vi "Select_List.vi"(7 "Load ERD List":T2) -> (8 "ERD Read List":T1(array[cluster])=[{"Boolean"=TRUE, "ERD Number"=49, "ERD Name"="Build Number", "Data Type"=enum."uint32_t"}, {"Boolean"=TRUE, "ERD Number"=127, "ERD Name"="Build Hash", "Data Type"=enum."string"}, {"Boolean"=TRUE, "ERD Number"=61467, "ERD Name"="Machine State", "Data Type"=enum."uint8_t"}, {"Boolean"=TRUE, "ERD Number"=61457, "ERD Name"="Relay Status", "Data Type"=enum."string"}, {"Boolean"=TRUE, "ERD Number"=61459, "ERD Name"="Door Switch State", "Data Type"=enum."string"}, {"Boolean"=TRUE, "ERD Number"=61460, "ERD Name"="Door Latch State", "Data Type"=enum."string"}, {"Boolean"=TRUE, "ERD Number"=61461, "ERD Name"="Inlet Thermistor", "Data Type"=enum."uint16_t"}, {"Boolean"=TRUE, "ERD Number"=61462, "ERD Name"="Outlet Thermistor", "Data Type"=enum."uint16_t"}, {"Boolean"=TRUE, "ERD Number"=61468, "ERD Name"="Control Lock State", "Data Type"=enum."string"}, {"Boolean"=TRUE, "ERD Number"=61483, "ERD Name"="Signal Volume", "Data Type"=enum."string"}, {"Boolean"=TRUE, "ERD Number"=61582, "ERD Name"="Drum Light", "Data Type"=enum."string"}, {"Boolean"=TRUE, "ERD Number"=61478, "ERD Name"="Delay Time", "Data Type"=enum."string"}, {"Boolean"=TRUE, "ERD Number"=8275, "ERD Name"="Ext. Tumble", "Data Type"=enum."string"}, {"Boolean"=TRUE, "ERD Number"=61480, "ERD Name"="Sub Cycle", "Data Type"=enum."uint8_t"}, {"Boolean"=TRUE, "ERD Number"=8272, "ERD Name"="Temp Level", "Data Type"=enum."string"}, {"Boolean"=TRUE, "ERD Number"=8269, "ERD Name"="Dryness Level", "Data Type"=enum."string"}, {"Boolean"=TRUE, "ERD Number"=8262, "ERD Name"="eDry", "Data Type"=enum."string"}, {"Boolean"=TRUE, "ERD Number"=61495, "ERD Name"="Time Level", "Data Type"=enum."string"}, {"Boolean"=TRUE, "ERD Number"=8266, "ERD Name"="Damp Alert", "Data Type"=enum."string"}, {"Boolean"=TRUE, "ERD Number"=61501, "ERD Name"="Detangle", "Data Type"=enum."string"}, {"Boolean"=TRUE, "ERD Number"=61510, "ERD Name"="MyCycle", "Data Type"=enum."string"}, {"Boolean"=TRUE, "ERD Number"=61594, "ERD Name"="Cycle Engine State", "Data Type"=enum."string"}, {"Boolean"=TRUE, "ERD Number"=61597, "ERD Name"="Cycle Selected", "Data Type"=enum."string"}, {"Boolean"=TRUE, "ERD Number"=61443, "ERD Name"="Tune ID", "Data Type"=enum."string"}, {"Boolean"=TRUE, "ERD Number"=61503, "ERD Name"="Delay Option", "Data Type"=enum."string"}, {"Boolean"=TRUE, "ERD Number"=61619, "ERD Name"="Restriction Detection Status", "Data Type"=enum."string"}, {"Boolean"=TRUE, "ERD Number"=61618, "ERD Name"="Vent Restriction", "Data Type"=enum."string"}, {"Boolean"=TRUE, "ERD Number"=61611, "ERD Name"="Load Size By Contact", "Data Type"=enum."string"}, {"Boolean"=TRUE, "ERD Number"=61613, "ERD Name"="Load Size by Temp", "Data Type"=enum."string"}, {"Boolean"=TRUE, "ERD Number"=61615, "ERD Name"="LoadSizeByAggregation", "Data Type"=enum."string"}, {"Boolean"=TRUE, "ERD Number"=61605, "ERD Name"="Sensor Dry Status", "Data Type"=enum."string"}, {"Boolean"=TRUE, "ERD Number"=61626, "ERD Name"="Check Dampness State", "Data Type"=enum."string"}, {"Boolean"=TRUE, "ERD Number"=61624, "ERD Name"="MoistureSensorRawAdcFromMc", "Data Type"=enum."string"}, {"Boolean"=TRUE, "ERD Number"=62242, "ERD Name"="SmoothMoistureReading", "Data Type"=enum."string"}, {"Boolean"=TRUE, "ERD Number"=61463, "ERD Name"="Filtered Moisture", "Data Type"=enum."string"}, {"Boolean"=TRUE, "ERD Number"=61608, "ERD Name"="TargetMoistureVoltage", "Data Type"=enum."string"}, {"Boolean"=TRUE, "ERD Number"=61609, "ERD Name"="TargetMoistureVoltageReached", "Data Type"=enum."string"}, {"Boolean"=TRUE, "ERD Number"=61719, "ERD Name"="MaxFilteredMoistureVoltageDuringASensingCycle", "Data Type"=enum."string"}, {"Boolean"=TRUE, "ERD Number"=61555, "ERD Name"="TrimmerBothCoilInhibitRequest", "Data Type"=enum."string"}, {"Boolean"=TRUE, "ERD Number"=61567, "ERD Name"="TrimmerInhibitRelay1", "Data Type"=enum."string"}, {"Boolean"=TRUE, "ERD Number"=61568, "ERD Name"="TrimmerInhibitRelay2", "Data Type"=enum."string"}, {"Boolean"=TRUE, "ERD Number"=61549, "ERD Name"="HeatControlParametricData", "Data Type"=enum."string"}, {"Boolean"=TRUE, "ERD Number"=61610, "ERD Name"="EOC Reason", "Data Type"=enum."string"}, {"Boolean"=TRUE, "ERD Number"=61600, "ERD Name"="Heat Control Request", "Data Type"=enum."string"}, {"Boolean"=TRUE, "ERD Number"=61677, "ERD Name"="CoolDownStepStatus", "Data Type"=enum."string"}, {"Boolean"=TRUE, "ERD Number"=61554, "ERD Name"="OverTempHeaterInhibitRequest", "Data Type"=enum."string"}, {"Boolean"=TRUE, "ERD Number"=61565, "ERD Name"="EcoDryInhibitRelay1", "Data Type"=enum."string"}, {"Boolean"=TRUE, "ERD Number"=61566, "ERD Name"="EcoDryInhibitRelay2", "Data Type"=enum."string"}, {"Boolean"=TRUE, "ERD Number"=61743, "ERD Name"="ReverseDrumInhibitRelay1", "Data Type"=enum."string"}, {"Boolean"=TRUE, "ERD Number"=61744, "ERD Name"="ReverseDrumInhibitRelay2", "Data Type"=enum."string"}, {"Boolean"=TRUE, "ERD Number"=61556, "ERD Name"="NormalHeatControlMethodStatus", "Data Type"=enum."string"}, {"Boolean"=TRUE, "ERD Number"=61557, "ERD Name"="FallbackHeatControlMethodStatus", "Data Type"=enum."string"}, {"Boolean"=TRUE, "ERD Number"=61479, "ERD Name"="Remaining Cycle Time", "Data Type"=enum."string"}, {"Boolean"=TRUE, "ERD Number"=61698, "ERD Name"="InitialHeatingCycleTimeSeconds", "Data Type"=enum."string"}, {"Boolean"=TRUE, "ERD Number"=62214, "ERD Name"="InletTemperatureRawAdc\n", "Data Type"=enum."string"}, {"Boolean"=TRUE, "ERD Number"=62215, "ERD Name"="OutletTemperatureRawAdc", "Data Type"=enum."string"}, {"Boolean"=TRUE, "ERD Number"=61607, "ERD Name"="SensingCycleTotalDryingTimeSeconds", "Data Type"=enum."string"}, {"Boolean"=TRUE, "ERD Number"=61563, "ERD Name"="TimedCycleTotalDryingTimeSeconds", "Data Type"=enum."string"}, {"Boolean"=TRUE, "ERD Number"=61628, "ERD Name"="TimeToReachTargetVoltageSeconds", "Data Type"=enum."string"}, {"Boolean"=TRUE, "ERD Number"=61617, "ERD Name"="Dry Load Detection", "Data Type"=enum."string"}, {"Boolean"=TRUE, "ERD Number"=63510, "ERD Name"="Sensor DryTemp Multiplier 100", "Data Type"=enum."string"}, {"Boolean"=TRUE, "ERD Number"=61728, "ERD Name"="Erd_EcoDrySensorDryProfileSelectorStatus", "Data Type"=enum."string"}, {"Boolean"=TRUE, "ERD Number"=61729, "ERD Name"="Erd_EcoDrySensorDryProfileSelectorResultmeInSeconds", "Data Type"=enum."string"}, {"Boolean"=TRUE, "ERD Number"=61736, "ERD Name"="Erd_EcoDryControllerStatus", "Data Type"=enum."string"}, {"Boolean"=TRUE, "ERD Number"=61737, "ERD Name"="Erd_EcoDryRelay1TimerData", "Data Type"=enum."string"}, {"Boolean"=TRUE, "ERD Number"=61738, "ERD Name"="Erd_EcoDryRelay2TimerData", "Data Type"=enum."string"}, {"Boolean"=TRUE, "ERD Number"=61739, "ERD Name"="Erd_EcoDryStage2TransitionTimeInSeconds", "Data Type"=enum."string"}, {"Boolean"=TRUE, "ERD Number"=61606, "ERD Name"="Erd_ElapsedCycleTimeSeconds2TransitionTimeInSeconds", "Data Type"=enum."string"}, {"Boolean"=TRUE, "ERD Number"=63489, "ERD Name"="SensorDryDampSmallRestrictionSmallLoad\natus", "Data Type"=enum."string"}] {"ERD Number" format="%.0x"})   [LabVIEW 2023]
uses:
  Common/type defs/Choose_ERD_List.ctl
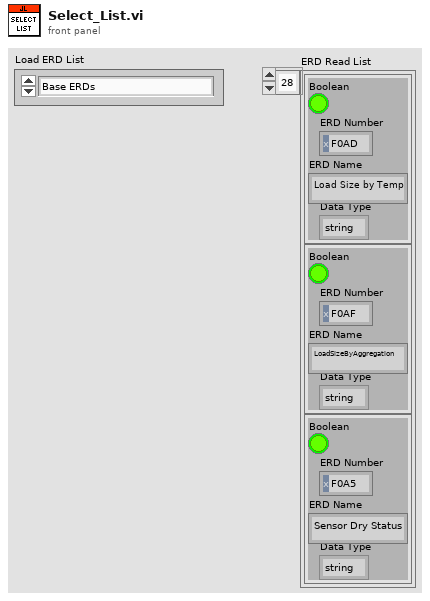
[diagram p1: front panel]
types:
  T1 = cluster{"Boolean":bool, "ERD Number":u16, "ERD Name":string, "Data Type":enum16{"string", "boolean", "uint8_t", "uint16_t", "uint32_t", "uint64_t", "int8_t", "int16_t", "int32_t", "int64_t"}}[]
  T2 = typedef "Choose_ERD_List.ctl" = enum16{"Base ERDs", "QA ERDs", "MABE ERD List", "EcoDry Evaluation ERD List", "ClothDampnessCheck ERD List"}
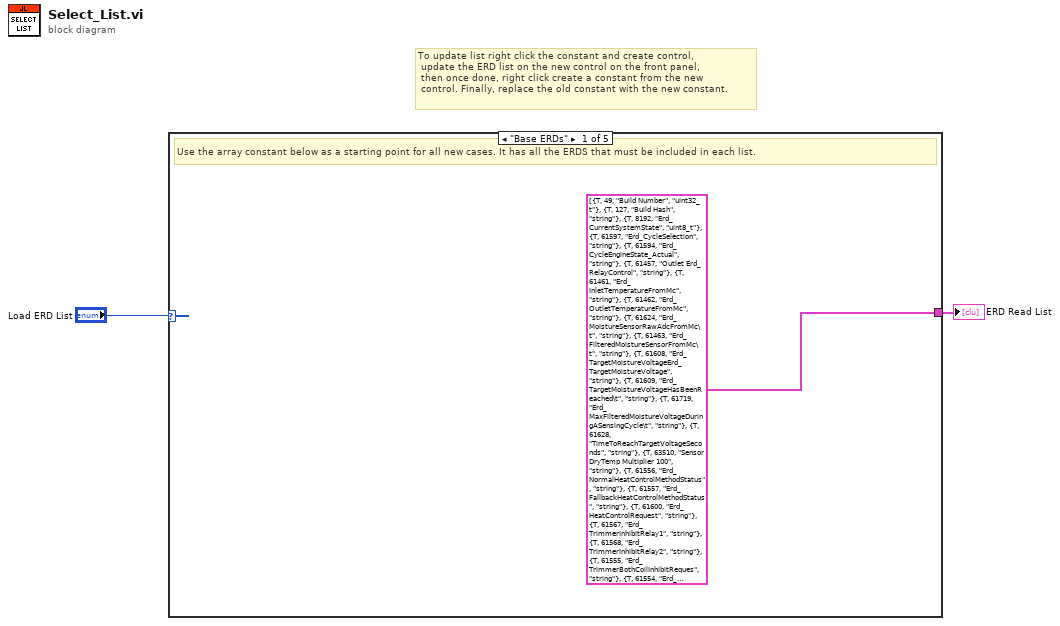
[diagram p0: block diagram]
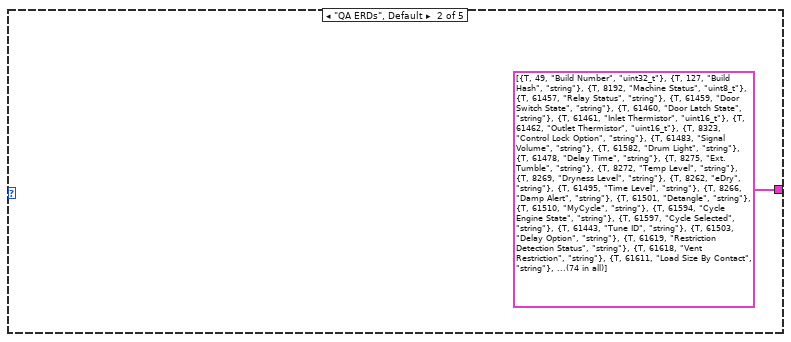
[diagram p2: hidden frame]
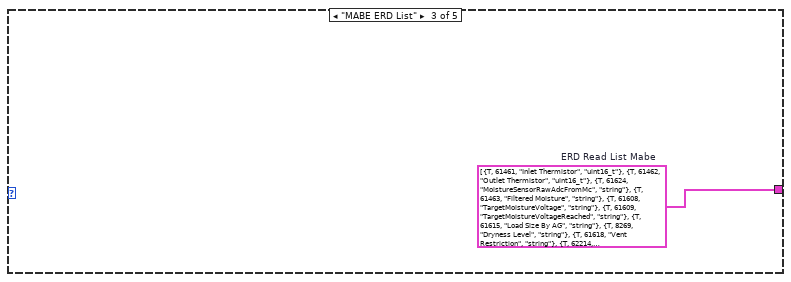
[diagram p3: hidden frame]
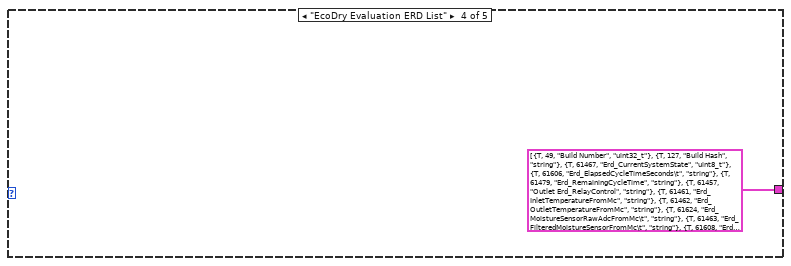
[diagram p4: hidden frame]
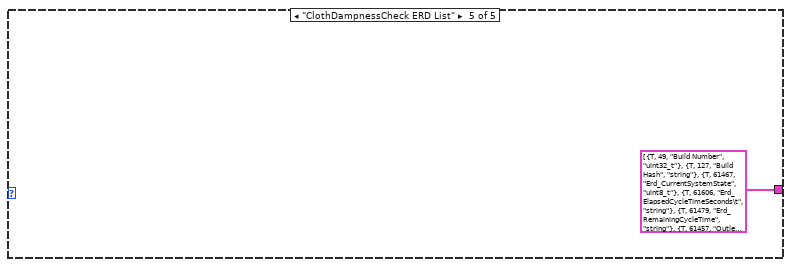
[diagram p5: hidden frame]
diagram:
  # "To update list right click the constant and create control,\n update the ERD list on the new control on the front panel,\n then once done, right click create a constant from the new\n control. Finally, replace the old constant with the new constant."
  n1 = case shown="\"Base ERDs\"" "Load ERD List" {
    tunnel: [T1 [{"Boolean"=TRUE, "ERD Number"=49, "ERD Name"="Build Number", "Data Type"=enum."uint32_t"}, {"Boolean"=TRUE, "ERD Number"=127, "ERD Name"="Build Hash", "Data Type"=enum."string"}, {"Boolean"=TRUE, "ERD Number"=8192, "ERD Name"="Erd_CurrentSystemState", "Data Type"=enum."uint8_t"}, {"Boolean"=TRUE, "ERD Number"=61597, "ERD Name"="Erd_CycleSelection", "Data Type"=enum."string"}, {"Boolean"=TRUE, "ERD Number"=61594, "ERD Name"="Erd_CycleEngineState_Actual", "Data Type"=enum."string"}, {"Boolean"=TRUE, "ERD Number"=61457, "ERD Name"="Outlet Erd_RelayControl", "Data Type"=enum."string"}, {"Boolean"=TRUE, "ERD Number"=61461, "ERD Name"="Erd_InletTemperatureFromMc", "Data Type"=enum."string"}, {"Boolean"=TRUE, "ERD Number"=61462, "ERD Name"="Erd_OutletTemperatureFromMc", "Data Type"=enum."string"}, {"Boolean"=TRUE, "ERD Number"=61624, "ERD Name"="Erd_MoistureSensorRawAdcFromMc\t", "Data Type"=enum."string"}, {"Boolean"=TRUE, "ERD Number"=61463, "ERD Name"="Erd_FilteredMoistureSensorFromMc\t", "Data Type"=enum."string"}, {"Boolean"=TRUE, "ERD Number"=61608, "ERD Name"="Erd_TargetMoistureVoltageErd_TargetMoistureVoltage", "Data Type"=enum."string"}, {"Boolean"=TRUE, "ERD Number"=61609, "ERD Name"="Erd_TargetMoistureVoltageHasBeenReached\t", "Data Type"=enum."string"}, {"Boolean"=TRUE, "ERD Number"=61719, "ERD Name"="Erd_MaxFilteredMoistureVoltageDuringASensingCycle\t", "Data Type"=enum."string"}, {"Boolean"=TRUE, "ERD Number"=61628, "ERD Name"="TimeToReachTargetVoltageSeconds", "Data Type"=enum."string"}, {"Boolean"=TRUE, "ERD Number"=63510, "ERD Name"="Sensor DryTemp Multiplier 100", "Data Type"=enum."string"}, {"Boolean"=TRUE, "ERD Number"=61556, "ERD Name"="Erd_NormalHeatControlMethodStatus", "Data Type"=enum."string"}, {"Boolean"=TRUE, "ERD Number"=61557, "ERD Name"="Erd_FallbackHeatControlMethodStatus", "Data Type"=enum."string"}, {"Boolean"=TRUE, "ERD Number"=61600, "ERD Name"="Erd_HeatControlRequest", "Data Type"=enum."string"}, {"Boolean"=TRUE, "ERD Number"=61567, "ERD Name"="Erd_TrimmerInhibitRelay1", "Data Type"=enum."string"}, {"Boolean"=TRUE, "ERD Number"=61568, "ERD Name"="Erd_TrimmerInhibitRelay2", "Data Type"=enum."string"}, {"Boolean"=TRUE, "ERD Number"=61555, "ERD Name"="Erd_TrimmerBothCoilInhibitReques", "Data Type"=enum."string"}, {"Boolean"=TRUE, "ERD Number"=61554, "ERD Name"="Erd_OverTempHeaterInhibitRequest", "Data Type"=enum."string"}, {"Boolean"=TRUE, "ERD Number"=61565, "ERD Name"="Erd_EcoDryInhibitRelay1", "Data Type"=enum."string"}, {"Boolean"=TRUE, "ERD Number"=61459, "ERD Name"="Erd_DoorIsClosed", "Data Type"=enum."string"}, {"Boolean"=TRUE, "ERD Number"=61463, "ERD Name"="Erd_FilteredMoistureSensorFromMc", "Data Type"=enum."string"}, {"Boolean"=TRUE, "ERD Number"=61457, "ERD Name"="Erd_RelayControl.drumMotor", "Data Type"=enum."string"}, {"Boolean"=TRUE, "ERD Number"=53, "ERD Name"="Erd_AppliancePersonality", "Data Type"=enum."string"}, {"Boolean"=TRUE, "ERD Number"=57, "ERD Name"="Erd_BootloaderVersion", "Data Type"=enum."string"}, {"Boolean"=TRUE, "ERD Number"=8311, "ERD Name"="Erd_TimeLevelOption", "Data Type"=enum."string"}, {"Boolean"=TRUE, "ERD Number"=8312, "ERD Name"="Erd_TimeLevelOptionRequest", "Data Type"=enum."string"}, {"Boolean"=TRUE, "ERD Number"=61479, "ERD Name"="Erd_RemainingCycleTime", "Data Type"=enum."string"}, {"Boolean"=TRUE, "ERD Number"=63489, "ERD Name"="Add Name", "Data Type"=enum."string"}] ("Base ERD list") T1 [{"Boolean"=TRUE, "ERD Number"=49, "ERD Name"="Build Number", "Data Type"=enum."uint32_t"}, {"Boolean"=TRUE, "ERD Number"=127, "ERD Name"="Build Hash", "Data Type"=enum."string"}, {"Boolean"=TRUE, "ERD Number"=8192, "ERD Name"="Machine Status", "Data Type"=enum."uint8_t"}, {"Boolean"=TRUE, "ERD Number"=61457, "ERD Name"="Relay Status", "Data Type"=enum."string"}, {"Boolean"=TRUE, "ERD Number"=61459, "ERD Name"="Door Switch State", "Data Type"=enum."string"}, {"Boolean"=TRUE, "ERD Number"=61460, "ERD Name"="Door Latch State", "Data Type"=enum."string"}, {"Boolean"=TRUE, "ERD Number"=61461, "ERD Name"="Inlet Thermistor", "Data Type"=enum."uint16_t"}, {"Boolean"=TRUE, "ERD Number"=61462, "ERD Name"="Outlet Thermistor", "Data Type"=enum."uint16_t"}, {"Boolean"=TRUE, "ERD Number"=8323, "ERD Name"="Control Lock Option", "Data Type"=enum."string"}, {"Boolean"=TRUE, "ERD Number"=61483, "ERD Name"="Signal Volume", "Data Type"=enum."string"}, {"Boolean"=TRUE, "ERD Number"=61582, "ERD Name"="Drum Light", "Data Type"=enum."string"}, {"Boolean"=TRUE, "ERD Number"=61478, "ERD Name"="Delay Time", "Data Type"=enum."string"}, {"Boolean"=TRUE, "ERD Number"=8275, "ERD Name"="Ext. Tumble", "Data Type"=enum."string"}, {"Boolean"=TRUE, "ERD Number"=8272, "ERD Name"="Temp Level", "Data Type"=enum."string"}, {"Boolean"=TRUE, "ERD Number"=8269, "ERD Name"="Dryness Level", "Data Type"=enum."string"}, {"Boolean"=TRUE, "ERD Number"=8262, "ERD Name"="eDry", "Data Type"=enum."string"}, {"Boolean"=TRUE, "ERD Number"=61495, "ERD Name"="Time Level", "Data Type"=enum."string"}, {"Boolean"=TRUE, "ERD Number"=8266, "ERD Name"="Damp Alert", "Data Type"=enum."string"}, {"Boolean"=TRUE, "ERD Number"=61501, "ERD Name"="Detangle", "Data Type"=enum."string"}, {"Boolean"=TRUE, "ERD Number"=61510, "ERD Name"="MyCycle", "Data Type"=enum."string"}, {"Boolean"=TRUE, "ERD Number"=61594, "ERD Name"="Cycle Engine State", "Data Type"=enum."string"}, {"Boolean"=TRUE, "ERD Number"=61597, "ERD Name"="Cycle Selected", "Data Type"=enum."string"}, {"Boolean"=TRUE, "ERD Number"=61443, "ERD Name"="Tune ID", "Data Type"=enum."string"}, {"Boolean"=TRUE, "ERD Number"=61503, "ERD Name"="Delay Option", "Data Type"=enum."string"}, {"Boolean"=TRUE, "ERD Number"=61619, "ERD Name"="Restriction Detection Status", "Data Type"=enum."string"}, {"Boolean"=TRUE, "ERD Number"=61618, "ERD Name"="Vent Restriction", "Data Type"=enum."string"}, {"Boolean"=TRUE, "ERD Number"=61611, "ERD Name"="Load Size By Contact", "Data Type"=enum."string"}, {"Boolean"=TRUE, "ERD Number"=61613, "ERD Name"="Load Size by Temp", "Data Type"=enum."string"}, {"Boolean"=TRUE, "ERD Number"=61615, "ERD Name"="LoadSizeByAggregation", "Data Type"=enum."string"}, {"Boolean"=TRUE, "ERD Number"=61605, "ERD Name"="Sensor Dry Status", "Data Type"=enum."string"}, {"Boolean"=TRUE, "ERD Number"=61626, "ERD Name"="Check Dampness State", "Data Type"=enum."string"}, {"Boolean"=TRUE, "ERD Number"=61624, "ERD Name"="MoistureSensorRawAdcFromMc", "Data Type"=enum."string"}, {"Boolean"=TRUE, "ERD Number"=62242, "ERD Name"="SmoothMoistureReading", "Data Type"=enum."string"}, {"Boolean"=TRUE, "ERD Number"=61463, "ERD Name"="Filtered Moisture", "Data Type"=enum."string"}, {"Boolean"=TRUE, "ERD Number"=61608, "ERD Name"="TargetMoistureVoltage", "Data Type"=enum."string"}, {"Boolean"=TRUE, "ERD Number"=61609, "ERD Name"="TargetMoistureVoltageReached", "Data Type"=enum."string"}, {"Boolean"=TRUE, "ERD Number"=61719, "ERD Name"="MaxFilteredMoistureVoltageDuringASensingCycle", "Data Type"=enum."string"}, {"Boolean"=TRUE, "ERD Number"=61555, "ERD Name"="TrimmerBothCoilInhibitRequest", "Data Type"=enum."string"}, {"Boolean"=TRUE, "ERD Number"=61567, "ERD Name"="TrimmerInhibitRelay1", "Data Type"=enum."string"}, {"Boolean"=TRUE, "ERD Number"=61568, "ERD Name"="TrimmerInhibitRelay2", "Data Type"=enum."string"}, {"Boolean"=TRUE, "ERD Number"=61549, "ERD Name"="HeatControlParametricData", "Data Type"=enum."string"}, {"Boolean"=TRUE, "ERD Number"=61610, "ERD Name"="EOC Reason", "Data Type"=enum."string"}, {"Boolean"=TRUE, "ERD Number"=61600, "ERD Name"="Heat Control Request", "Data Type"=enum."string"}, {"Boolean"=TRUE, "ERD Number"=61677, "ERD Name"="CoolDownStepStatus", "Data Type"=enum."string"}, {"Boolean"=TRUE, "ERD Number"=61554, "ERD Name"="OverTempHeaterInhibitRequest", "Data Type"=enum."string"}, {"Boolean"=TRUE, "ERD Number"=61565, "ERD Name"="EcoDryInhibitRelay1", "Data Type"=enum."string"}, {"Boolean"=TRUE, "ERD Number"=61566, "ERD Name"="EcoDryInhibitRelay2", "Data Type"=enum."string"}, {"Boolean"=TRUE, "ERD Number"=61743, "ERD Name"="ReverseDrumInhibitRelay1", "Data Type"=enum."string"}, {"Boolean"=TRUE, "ERD Number"=61744, "ERD Name"="ReverseDrumInhibitRelay2", "Data Type"=enum."string"}, {"Boolean"=TRUE, "ERD Number"=61556, "ERD Name"="NormalHeatControlMethodStatus", "Data Type"=enum."string"}, {"Boolean"=TRUE, "ERD Number"=61557, "ERD Name"="FallbackHeatControlMethodStatus", "Data Type"=enum."string"}, {"Boolean"=TRUE, "ERD Number"=61479, "ERD Name"="Remaining Cycle Time", "Data Type"=enum."string"}, {"Boolean"=TRUE, "ERD Number"=61698, "ERD Name"="InitialHeatingCycleTimeSeconds", "Data Type"=enum."string"}, {"Boolean"=TRUE, "ERD Number"=62214, "ERD Name"="InletTemperatureRawAdc\n", "Data Type"=enum."string"}, {"Boolean"=TRUE, "ERD Number"=62215, "ERD Name"="OutletTemperatureRawAdc", "Data Type"=enum."string"}, {"Boolean"=TRUE, "ERD Number"=61607, "ERD Name"="SensingCycleTotalDryingTimeSeconds", "Data Type"=enum."string"}, {"Boolean"=TRUE, "ERD Number"=61563, "ERD Name"="TimedCycleTotalDryingTimeSeconds", "Data Type"=enum."string"}, {"Boolean"=TRUE, "ERD Number"=61628, "ERD Name"="TimeToReachTargetVoltageSeconds", "Data Type"=enum."string"}, {"Boolean"=TRUE, "ERD Number"=61617, "ERD Name"="Dry Load Detection", "Data Type"=enum."string"}, {"Boolean"=TRUE, "ERD Number"=63510, "ERD Name"="Sensor DryTemp Multiplier 100", "Data Type"=enum."string"}, {"Boolean"=TRUE, "ERD Number"=61728, "ERD Name"="Erd_EcoDrySensorDryProfileSelectorStatus", "Data Type"=enum."string"}, {"Boolean"=TRUE, "ERD Number"=61729, "ERD Name"="Erd_EcoDrySensorDryProfileSelectorResultmeInSeconds", "Data Type"=enum."string"}, {"Boolean"=TRUE, "ERD Number"=61736, "ERD Name"="Erd_EcoDryControllerStatus", "Data Type"=enum."string"}, {"Boolean"=TRUE, "ERD Number"=61737, "ERD Name"="Erd_EcoDryRelay1TimerData", "Data Type"=enum."string"}, {"Boolean"=TRUE, "ERD Number"=61738, "ERD Name"="Erd_EcoDryRelay2TimerData", "Data Type"=enum."string"}, {"Boolean"=TRUE, "ERD Number"=61739, "ERD Name"="Erd_EcoDryStage2TransitionTimeInSeconds", "Data Type"=enum."string"}, {"Boolean"=TRUE, "ERD Number"=8193, "ERD Name"="Erd_MachineSubCycle", "Data Type"=enum."string"}, {"Boolean"=TRUE, "ERD Number"=61606, "ERD Name"="Erd_ElapsedCycleTimeSeconds2TransitionTimeInSeconds", "Data Type"=enum."string"}, {"Boolean"=TRUE, "ERD Number"=58, "ERD Name"="Erd_ApplicationVersionallLoad\natus", "Data Type"=enum."string"}, {"Boolean"=TRUE, "ERD Number"=59, "ERD Name"="ParametricVersion", "Data Type"=enum."string"}, {"Boolean"=TRUE, "ERD Number"=57, "ERD Name"="Erd_BootloaderVersion", "Data Type"=enum."string"}, {"Boolean"=TRUE, "ERD Number"=8272, "ERD Name"="Erd_TemperatureOption", "Data Type"=enum."string"}, {"Boolean"=TRUE, "ERD Number"=8311, "ERD Name"="Erd_TimeLevelOption", "Data Type"=enum."string"}, {"Boolean"=TRUE, "ERD Number"=8192, "ERD Name"="SensorDryDampSmallRestrictionSmSeconds", "Data Type"=enum."string"}] ("QA ERDs") w5 T1 [{"Boolean"=TRUE, "ERD Number"=49, "ERD Name"="Build Number", "Data Type"=enum."uint32_t"}, {"Boolean"=TRUE, "ERD Number"=127, "ERD Name"="Build Hash", "Data Type"=enum."string"}, {"Boolean"=TRUE, "ERD Number"=61467, "ERD Name"="Erd_CurrentSystemState", "Data Type"=enum."uint8_t"}, {"Boolean"=TRUE, "ERD Number"=61606, "ERD Name"="Erd_ElapsedCycleTimeSeconds\t", "Data Type"=enum."string"}, {"Boolean"=TRUE, "ERD Number"=61479, "ERD Name"="Erd_RemainingCycleTime", "Data Type"=enum."string"}, {"Boolean"=TRUE, "ERD Number"=61457, "ERD Name"="Outlet Erd_RelayControl", "Data Type"=enum."string"}, {"Boolean"=TRUE, "ERD Number"=61461, "ERD Name"="Erd_InletTemperatureFromMc", "Data Type"=enum."string"}, {"Boolean"=TRUE, "ERD Number"=61462, "ERD Name"="Erd_OutletTemperatureFromMc", "Data Type"=enum."string"}, {"Boolean"=TRUE, "ERD Number"=61624, "ERD Name"="Erd_MoistureSensorRawAdcFromMc\t", "Data Type"=enum."string"}, {"Boolean"=TRUE, "ERD Number"=61463, "ERD Name"="Erd_FilteredMoistureSensorFromMc\t", "Data Type"=enum."string"}, {"Boolean"=TRUE, "ERD Number"=61608, "ERD Name"="Erd_TargetMoistureVoltageErd_TargetMoistureVoltage", "Data Type"=enum."string"}, {"Boolean"=TRUE, "ERD Number"=61609, "ERD Name"="Erd_TargetMoistureVoltageHasBeenReached\t", "Data Type"=enum."string"}, {"Boolean"=TRUE, "ERD Number"=61719, "ERD Name"="Erd_MaxFilteredMoistureVoltageDuringASensingCycle\t", "Data Type"=enum."string"}, {"Boolean"=TRUE, "ERD Number"=61628, "ERD Name"="TimeToReachTargetVoltageSeconds", "Data Type"=enum."string"}, {"Boolean"=TRUE, "ERD Number"=63510, "ERD Name"="Sensor DryTemp Multiplier 100", "Data Type"=enum."string"}, {"Boolean"=TRUE, "ERD Number"=61605, "ERD Name"="Erd_SensorDryStatus", "Data Type"=enum."string"}, {"Boolean"=TRUE, "ERD Number"=61607, "ERD Name"="Erd_SensingCycleTotalDryingTimeSeconds", "Data Type"=enum."string"}, {"Boolean"=TRUE, "ERD Number"=63074, "ERD Name"="Erd_EcoDryStage2DurationSeconds", "Data Type"=enum."string"}, {"Boolean"=TRUE, "ERD Number"=63075, "ERD Name"="Erd_EcoDryStage1PeriodSeconds", "Data Type"=enum."string"}, {"Boolean"=TRUE, "ERD Number"=63076, "ERD Name"="Erd_EcoDryStage1Heater1ActiveSeconds", "Data Type"=enum."string"}, {"Boolean"=TRUE, "ERD Number"=63077, "ERD Name"="Erd_EcoDryStage1Heater2ActiveSeconds", "Data Type"=enum."string"}, {"Boolean"=TRUE, "ERD Number"=63078, "ERD Name"="Erd_EcoDryStage2PeriodSeconds", "Data Type"=enum."string"}, {"Boolean"=TRUE, "ERD Number"=63079, "ERD Name"="Erd_EcoDryStage2Heater1ActiveSeconds", "Data Type"=enum."string"}, {"Boolean"=TRUE, "ERD Number"=63080, "ERD Name"="Erd_EcoDryStage2Heater2ActiveSeconds", "Data Type"=enum."string"}, {"Boolean"=TRUE, "ERD Number"=61736, "ERD Name"="Erd_EcoDryControllerStatus", "Data Type"=enum."string"}, {"Boolean"=TRUE, "ERD Number"=61737, "ERD Name"="Erd_EcoDryRelay1TimerData", "Data Type"=enum."string"}, {"Boolean"=TRUE, "ERD Number"=61738, "ERD Name"="Erd_EcoDryRelay2TimerData", "Data Type"=enum."string"}, {"Boolean"=TRUE, "ERD Number"=61739, "ERD Name"="Erd_EcoDryStage2TransitionTimeInSeconds", "Data Type"=enum."string"}, {"Boolean"=TRUE, "ERD Number"=61554, "ERD Name"="Erd_OverTempHeaterInhibitRequest", "Data Type"=enum."string"}, {"Boolean"=TRUE, "ERD Number"=61555, "ERD Name"="Erd_TrimmerBothCoilInhibitRequest", "Data Type"=enum."string"}, {"Boolean"=TRUE, "ERD Number"=61565, "ERD Name"="Erd_EcoDryInhibitRelay1", "Data Type"=enum."string"}, {"Boolean"=TRUE, "ERD Number"=61566, "ERD Name"="Erd_EcoDryInhibitRelay2", "Data Type"=enum."string"}, {"Boolean"=TRUE, "ERD Number"=61567, "ERD Name"="Erd_TrimmerInhibitRelay1", "Data Type"=enum."string"}, {"Boolean"=TRUE, "ERD Number"=61568, "ERD Name"="Erd_TrimmerInhibitRelay2\t", "Data Type"=enum."string"}, {"Boolean"=TRUE, "ERD Number"=61683, "ERD Name"="Erd_SteamHeatInhibitRelay1", "Data Type"=enum."string"}, {"Boolean"=TRUE, "ERD Number"=61684, "ERD Name"="Erd_SteamHeatInhibitRelay2\t", "Data Type"=enum."string"}, {"Boolean"=TRUE, "ERD Number"=61743, "ERD Name"="Erd_ReverseDrumInhibitRelay1\t", "Data Type"=enum."string"}, {"Boolean"=TRUE, "ERD Number"=61744, "ERD Name"="Erd_ReverseDrumInhibitRelay2\t", "Data Type"=enum."string"}, {"Boolean"=TRUE, "ERD Number"=63489, "ERD Name"="SensorDryDampSmallRestrictionSmallLoad\natus", "Data Type"=enum."string"}] ("Base ERD List Array Constant 2") T1 [{"Boolean"=TRUE, "ERD Number"=49, "ERD Name"="Build Number", "Data Type"=enum."uint32_t"}, {"Boolean"=TRUE, "ERD Number"=127, "ERD Name"="Build Hash", "Data Type"=enum."string"}, {"Boolean"=TRUE, "ERD Number"=61467, "ERD Name"="Erd_CurrentSystemState", "Data Type"=enum."uint8_t"}, {"Boolean"=TRUE, "ERD Number"=61606, "ERD Name"="Erd_ElapsedCycleTimeSeconds\t", "Data Type"=enum."string"}, {"Boolean"=TRUE, "ERD Number"=61479, "ERD Name"="Erd_RemainingCycleTime", "Data Type"=enum."string"}, {"Boolean"=TRUE, "ERD Number"=61457, "ERD Name"="Outlet Erd_RelayControl", "Data Type"=enum."string"}, {"Boolean"=TRUE, "ERD Number"=61461, "ERD Name"="Erd_InletTemperatureFromMc", "Data Type"=enum."string"}, {"Boolean"=TRUE, "ERD Number"=61462, "ERD Name"="Erd_OutletTemperatureFromMc", "Data Type"=enum."string"}, {"Boolean"=TRUE, "ERD Number"=61624, "ERD Name"="Erd_MoistureSensorRawAdcFromMc\t", "Data Type"=enum."string"}, {"Boolean"=TRUE, "ERD Number"=61463, "ERD Name"="Erd_FilteredMoistureSensorFromMc\t", "Data Type"=enum."string"}, {"Boolean"=TRUE, "ERD Number"=61608, "ERD Name"="Erd_TargetMoistureVoltageErd_TargetMoistureVoltage", "Data Type"=enum."string"}, {"Boolean"=TRUE, "ERD Number"=61609, "ERD Name"="Erd_TargetMoistureVoltageHasBeenReached\t", "Data Type"=enum."string"}, {"Boolean"=TRUE, "ERD Number"=61719, "ERD Name"="Erd_MaxFilteredMoistureVoltageDuringASensingCycle\t", "Data Type"=enum."string"}, {"Boolean"=TRUE, "ERD Number"=61628, "ERD Name"="TimeToReachTargetVoltageSeconds", "Data Type"=enum."string"}, {"Boolean"=TRUE, "ERD Number"=63510, "ERD Name"="Sensor DryTemp Multiplier 100", "Data Type"=enum."string"}, {"Boolean"=TRUE, "ERD Number"=61605, "ERD Name"="Erd_SensorDryStepStatus", "Data Type"=enum."string"}, {"Boolean"=TRUE, "ERD Number"=61481, "ERD Name"="Erd_CurrentDrynessState", "Data Type"=enum."string"}, {"Boolean"=TRUE, "ERD Number"=61626, "ERD Name"="Erd_ClothDampnessCheckResult", "Data Type"=enum."string"}, {"Boolean"=TRUE, "ERD Number"=61607, "ERD Name"="Erd_SensingCycleTotalDryingTimeSeconds", "Data Type"=enum."string"}, {"Boolean"=TRUE, "ERD Number"=61734, "ERD Name"="Erd_SensorDryDataSourceIndexKey", "Data Type"=enum."string"}, {"Boolean"=TRUE, "ERD Number"=8262, "ERD Name"="Erd_EcoDryOption", "Data Type"=enum."string"}, {"Boolean"=TRUE, "ERD Number"=8272, "ERD Name"="Erd_TemperatureOption", "Data Type"=enum."string"}, {"Boolean"=TRUE, "ERD Number"=8269, "ERD Name"="Erd_DrynessOption", "Data Type"=enum."string"}, {"Boolean"=TRUE, "ERD Number"=61618, "ERD Name"="Erd_VentRestriction", "Data Type"=enum."string"}, {"Boolean"=TRUE, "ERD Number"=63257, "ERD Name"="Erd_SanitizeOutletTempAdder", "Data Type"=enum."string"}, {"Boolean"=TRUE, "ERD Number"=63081, "ERD Name"="Erd_SanitizeMaxDryTimeInSeconds", "Data Type"=enum."string"}, {"Boolean"=TRUE, "ERD Number"=63258, "ERD Name"="Erd_SanitizeTimeAdderInSeconds", "Data Type"=enum."string"}, {"Boolean"=TRUE, "ERD Number"=61615, "ERD Name"="Erd_LoadSizeByAggregation", "Data Type"=enum."string"}, {"Boolean"=TRUE, "ERD Number"=63509, "ERD Name"="Erd_SensorDryMaxDryTimeSeconds", "Data Type"=enum."string"}, {"Boolean"=TRUE, "ERD Number"=63263, "ERD Name"="Erd_RequiresRestrictionAndLoadDetectionOnSensorDryCycles", "Data Type"=enum."string"}, {"Boolean"=TRUE, "ERD Number"=63489, "ERD Name"="SensorDryDampSmallRestrictionSmallLoad\natus", "Data Type"=enum."string"}] ("Base ERD List Array Constant 2")] -> w1
    frame "Base ERDs" {
      # "Use the array constant below as a starting point for all new cases. It has all the ERDS that must be included in each list."
    }
    frame "QA ERDs", Default {
    }
    frame "MABE ERD List" {
      w5 = T1 [{"Boolean"=TRUE, "ERD Number"=61461, "ERD Name"="Inlet Thermistor", "Data Type"=enum."uint16_t"}, {"Boolean"=TRUE, "ERD Number"=61462, "ERD Name"="Outlet Thermistor", "Data Type"=enum."uint16_t"}, {"Boolean"=TRUE, "ERD Number"=61624, "ERD Name"="MoistureSensorRawAdcFromMc", "Data Type"=enum."string"}, {"Boolean"=TRUE, "ERD Number"=61463, "ERD Name"="Filtered Moisture", "Data Type"=enum."string"}, {"Boolean"=TRUE, "ERD Number"=61608, "ERD Name"="TargetMoistureVoltage", "Data Type"=enum."string"}, {"Boolean"=TRUE, "ERD Number"=61609, "ERD Name"="TargetMoistureVoltageReached", "Data Type"=enum."string"}, {"Boolean"=TRUE, "ERD Number"=61615, "ERD Name"="Load Size By AG", "Data Type"=enum."string"}, {"Boolean"=TRUE, "ERD Number"=8269, "ERD Name"="Dryness Level", "Data Type"=enum."string"}, {"Boolean"=TRUE, "ERD Number"=61618, "ERD Name"="Vent Restriction", "Data Type"=enum."string"}, {"Boolean"=TRUE, "ERD Number"=62214, "ERD Name"="InletTemperatureRawAdc\n", "Data Type"=enum."string"}, {"Boolean"=TRUE, "ERD Number"=62215, "ERD Name"="OutletTemperatureRawAdc", "Data Type"=enum."string"}, {"Boolean"=TRUE, "ERD Number"=61628, "ERD Name"="TimeToReachTargetVoltageSeconds", "Data Type"=enum."string"}, {"Boolean"=TRUE, "ERD Number"=61607, "ERD Name"="SensingCycleTotalDryingTimeSeconds", "Data Type"=enum."string"}, {"Boolean"=TRUE, "ERD Number"=61457, "ERD Name"="Erd_RelayControl", "Data Type"=enum."string"}, {"Boolean"=TRUE, "ERD Number"=61719, "ERD Name"="Erd_MaxFilteredMoistureVoltageDuringASensingCycle\t", "Data Type"=enum."string"}, {"Boolean"=TRUE, "ERD Number"=61467, "ERD Name"="Erd_CurrentSystemState", "Data Type"=enum."string"}, {"Boolean"=TRUE, "ERD Number"=61606, "ERD Name"="Erd_ElapsedCycleTimeSecondsErd_ElapsedCycleTimeSeconds", "Data Type"=enum."string"}, {"Boolean"=TRUE, "ERD Number"=61479, "ERD Name"="Erd_RemainingCycleTime", "Data Type"=enum."string"}, {"Boolean"=TRUE, "ERD Number"=63510, "ERD Name"="Sensor DryTemp Multiplier 100", "Data Type"=enum."string"}, {"Boolean"=TRUE, "ERD Number"=63489, "ERD Name"="SensorDryDampSmallRestrictionSmallLoad\natus", "Data Type"=enum."string"}]  # ERD Read List Mabe
    }
    frame "EcoDry Evaluation ERD List" {
    }
    frame "ClothDampnessCheck ERD List" {
    }
  }
  "ERD Read List" <- w1
